vi "SET_EXCIT_LEVEL_n.vi"(2 "execute":bool, 7 "Level":u32 max=255 step=1, 11 "error in (no error)":errorcluster) -> (4 "function return":string, 15 "error out":errorcluster)   [LabVIEW 2017, in "ZBOX_IS.lvlib"]
uses:
  ZBOX_IS.lvlib
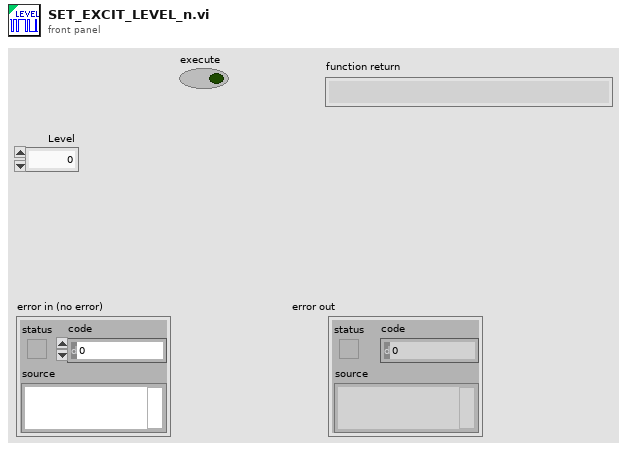
[diagram p1: front panel]
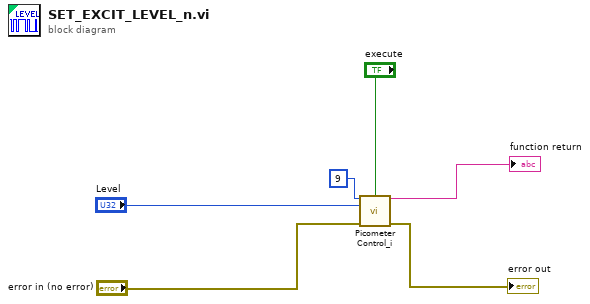
[diagram p0: block diagram]
diagram:
  n1 = call "Picometer Control_i.vi"("Cmd"=u8 9, "execute"="execute", "ulValue"="Level", "error in (no error)"="error in (no error)") -> ("function return"=→"function return":string, "error out"=→"error out":errorcluster)  [unwired: 7 in, 3 out]
